vi "NMR only mode.vi"() -> ()   [LabVIEW 2010]
uses:
  QCA-Q_Curve_Acquisition/QCA Global.vi
panel:
  in  "setup\nfile":path=path "C:/Users/ptgroup/Documents/PDP/B28_Setup_File.txt"
  in  "DC convert":bool
  in  "DAC channel":u32
  in  "ADC channel":u32=1 step=1
  in  "Q meter number":u32=2 step=1
  out "update in (s)":u32
  in  "run":bool
  in  "single shot":bool
  in  "Yale gain":u16(ring)=1 items=["1", "20", "50"]
  in  "sweeps":u32=100
  in  "steps / second":u32=15287 step=1
  in  "steps":u32=500 step=1
  in  "amplitude (mV)":i32=275
  in  "modulation (kHz)":i32=400 step=1
  in  "center frequency (MHz)":dbl=213.0 min=0.0 step=0.001 format="%#_6f"
  out "NMR signal":cluster{dbl[], "Waveform Graph":dbl[]}(graph)
  # "RF settings"
  # "sweep settings"
  # "Q meter settings"
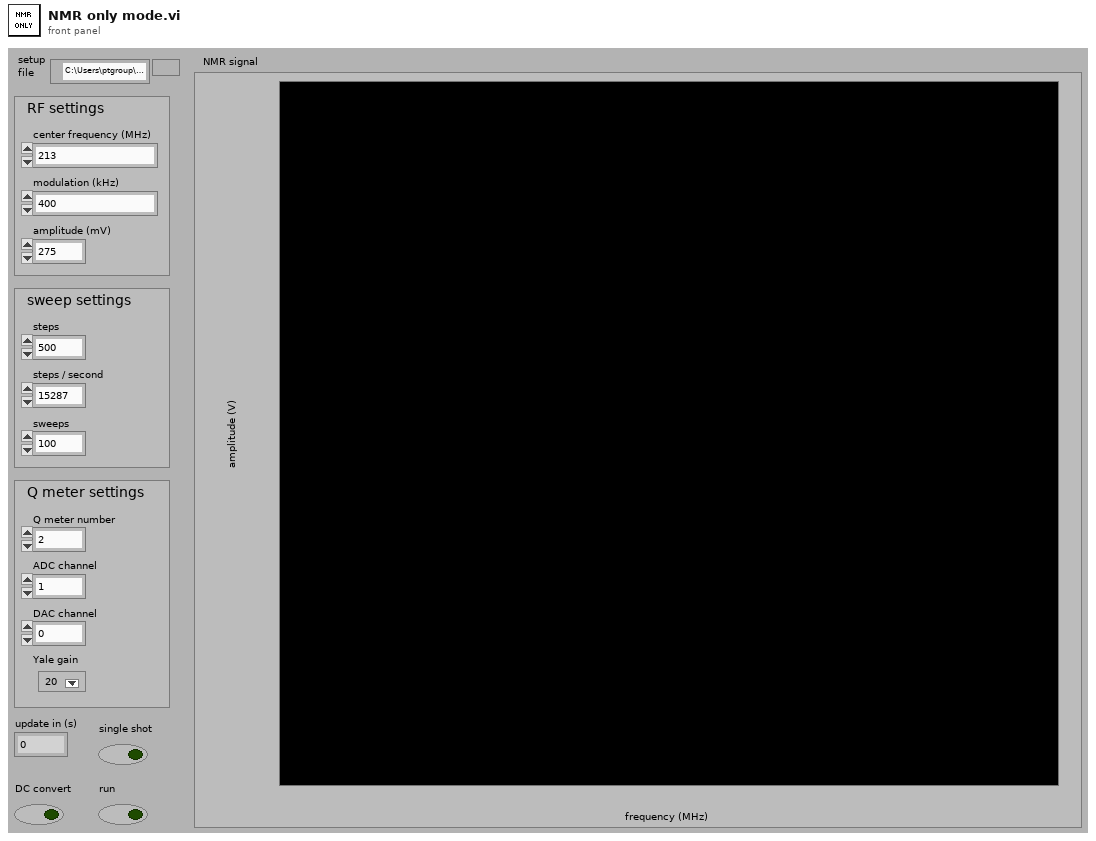
[diagram p1: front panel]
types:
  T1 = enum16{"initialize TPS", "initialize NMR", "initialize RF", "initialize Yale", "idle", "run", "single shot", "stop"}
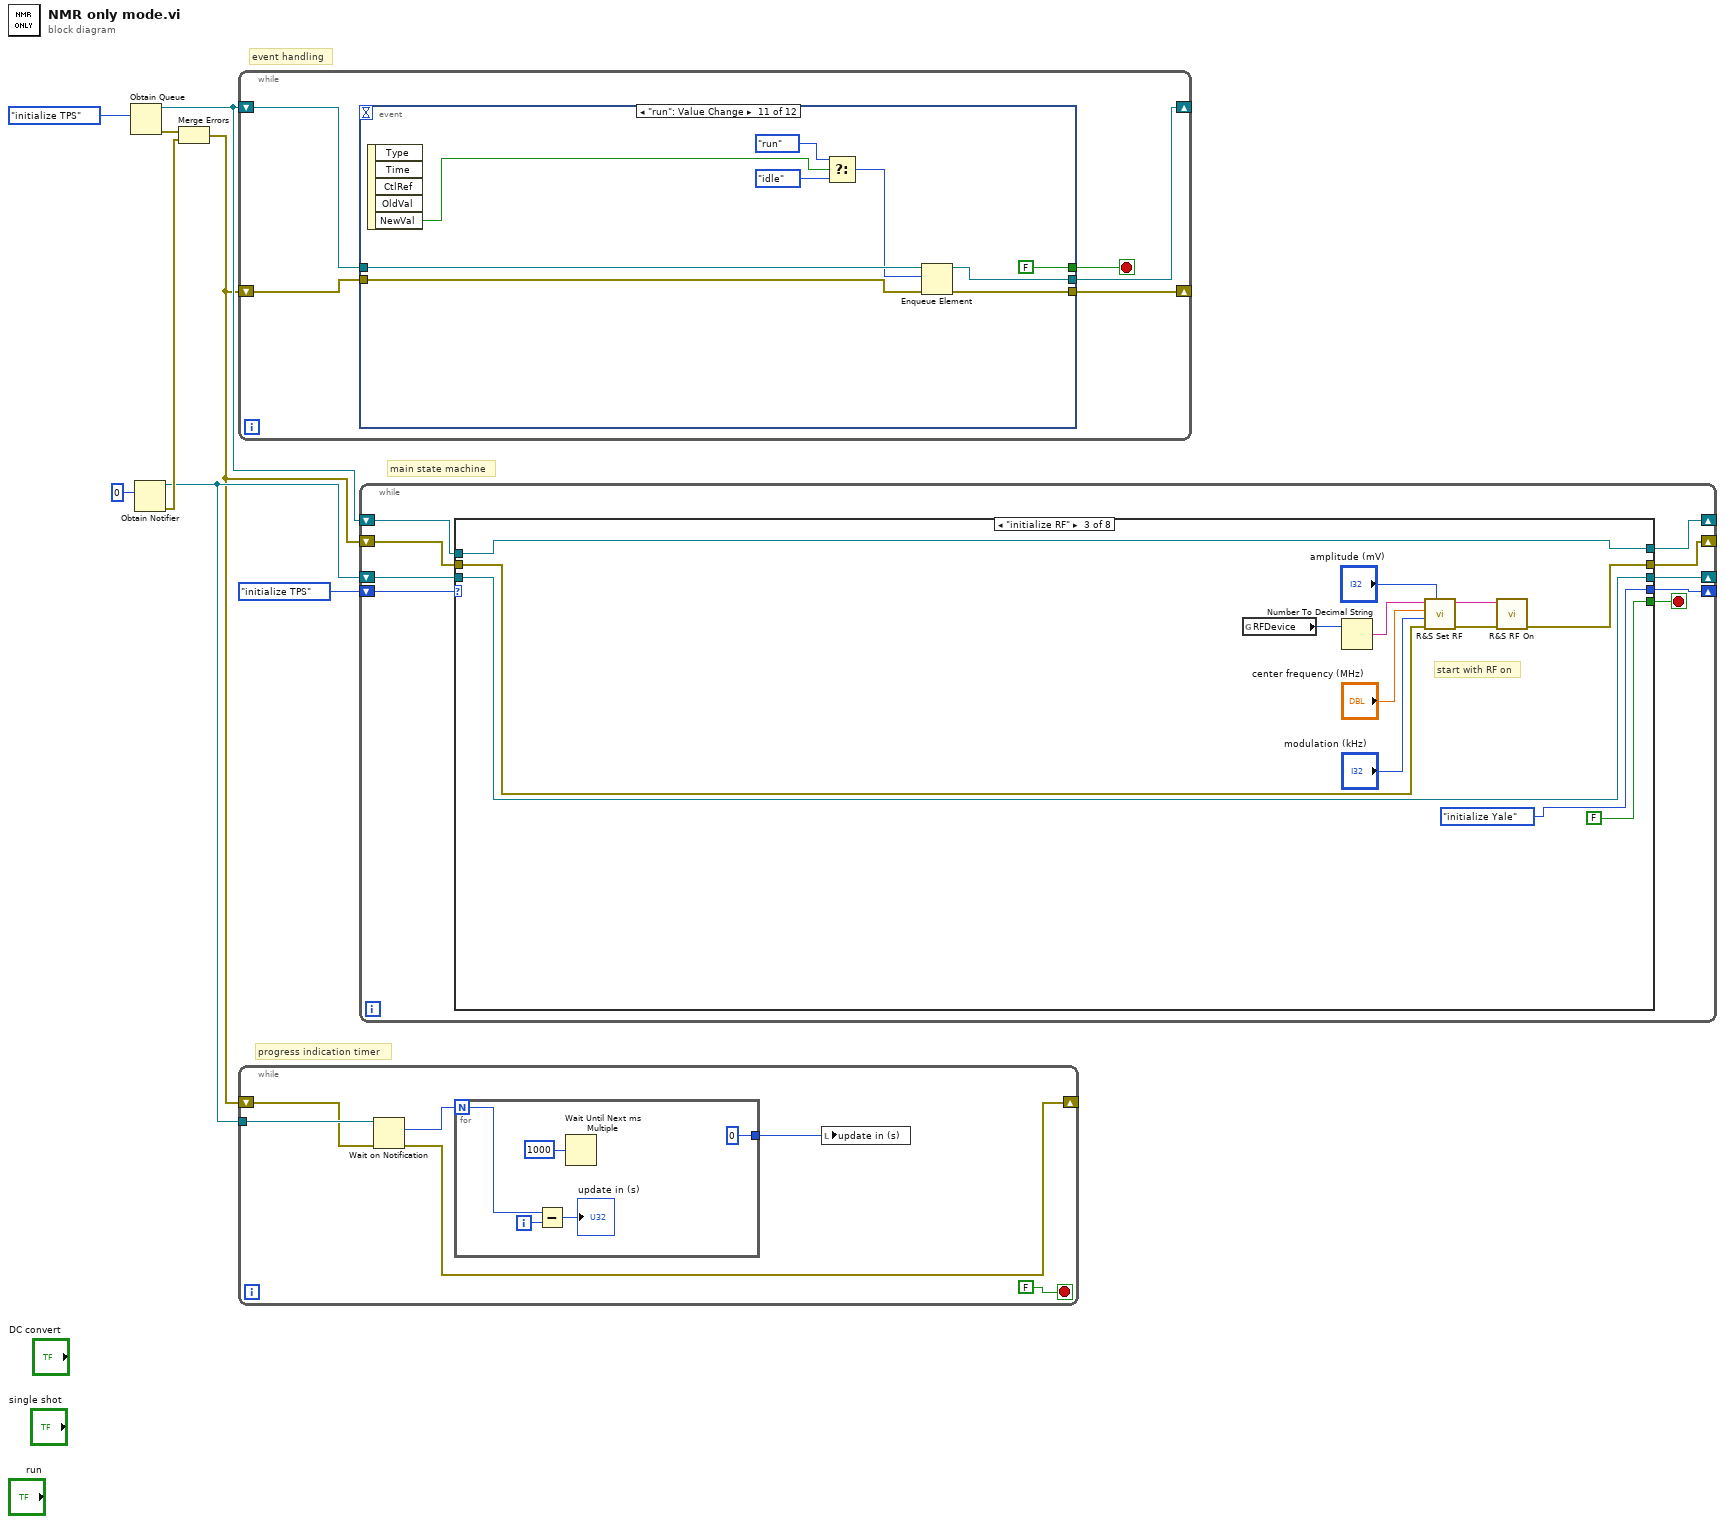
[diagram p0: block diagram]
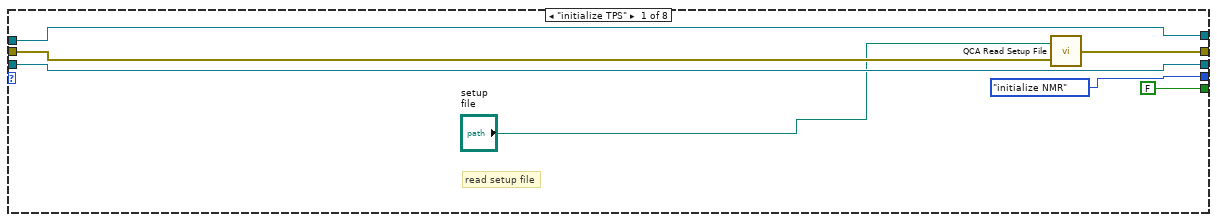
[diagram p2: hidden frame]
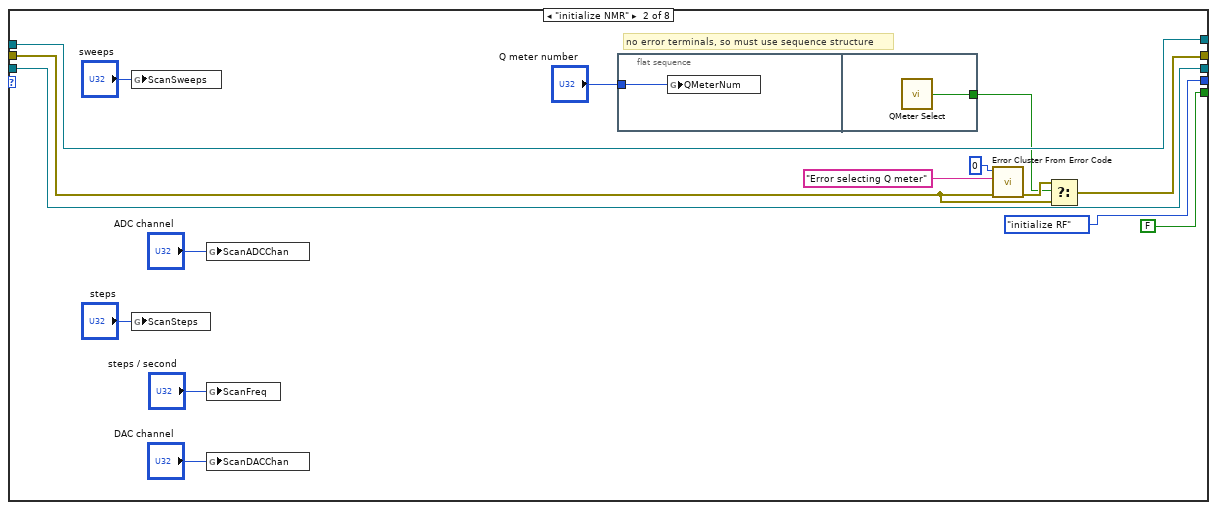
[diagram p3: hidden frame]
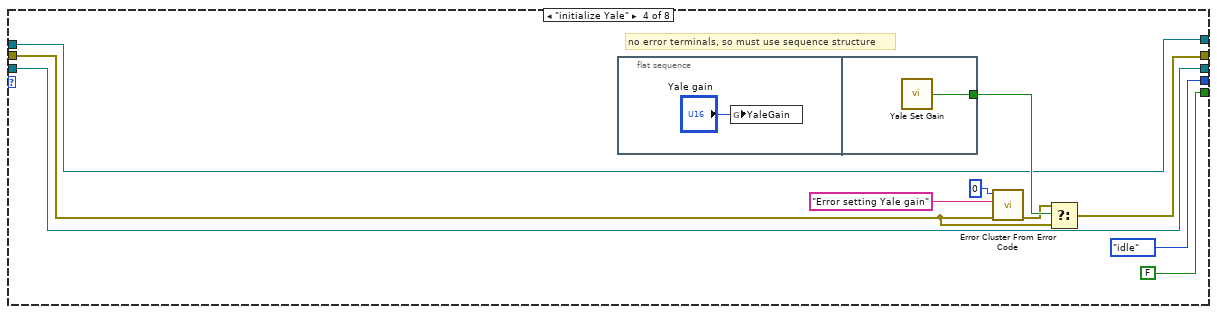
[diagram p4: hidden frame]
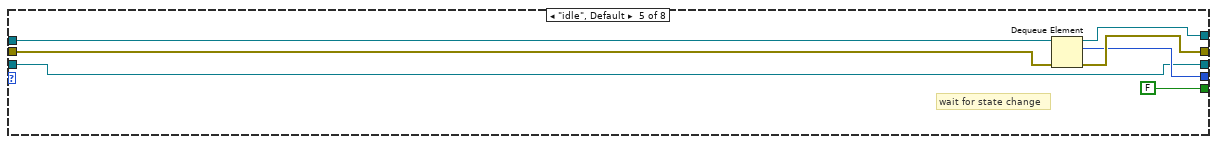
[diagram p5: hidden frame]
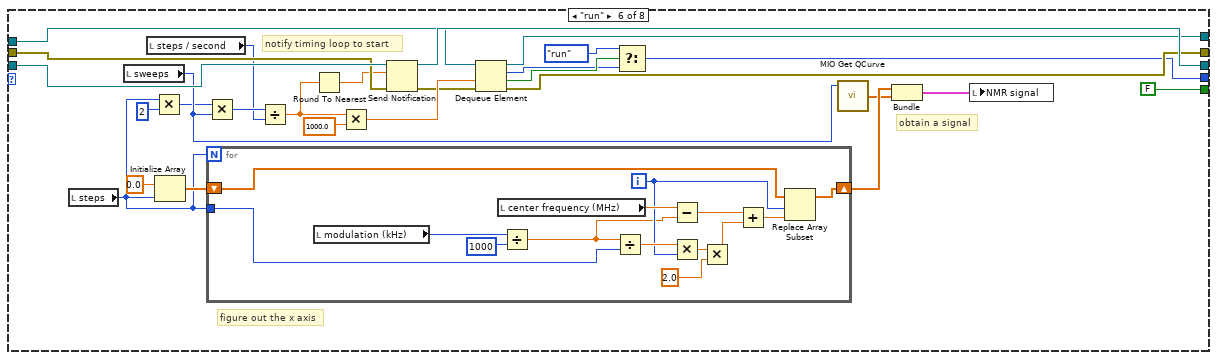
[diagram p6: hidden frame]
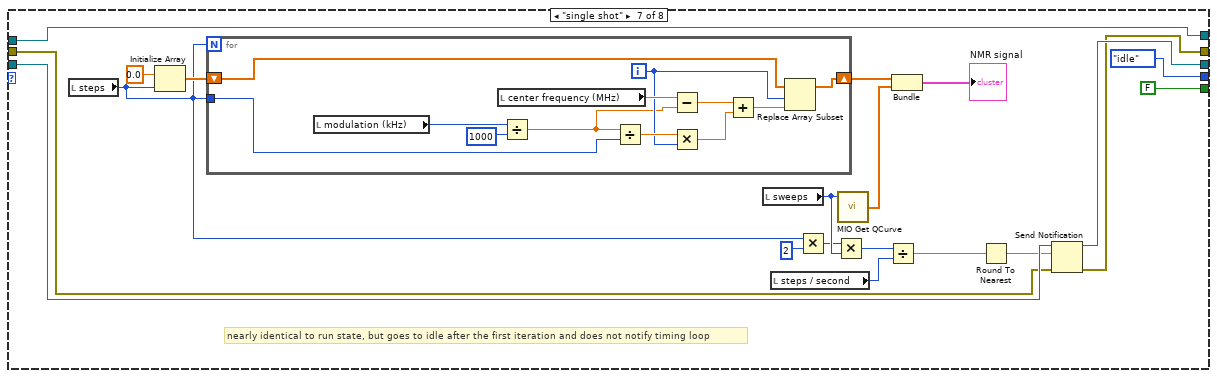
[diagram p7: hidden frame]
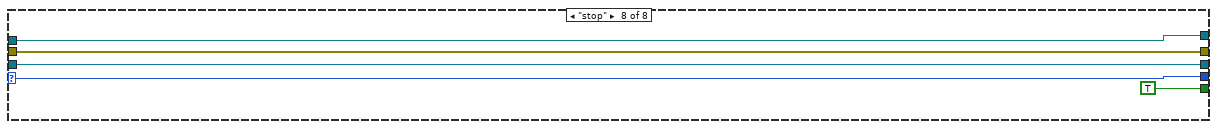
[diagram p8: hidden frame]
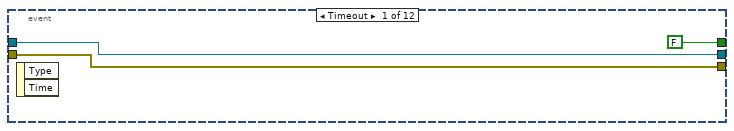
[diagram p9: hidden frame]
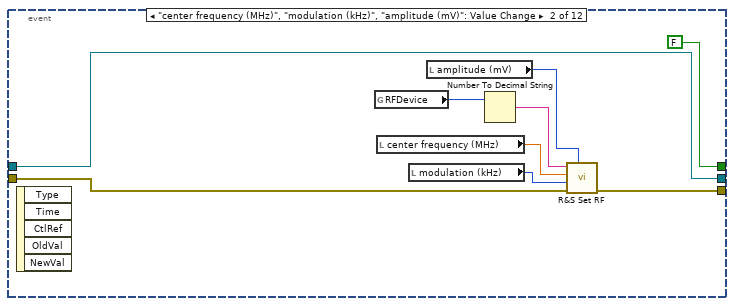
[diagram p10: hidden frame]
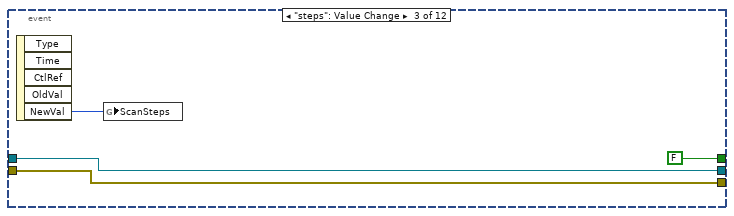
[diagram p11: hidden frame]
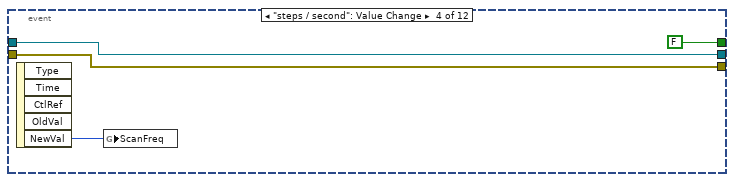
[diagram p12: hidden frame]
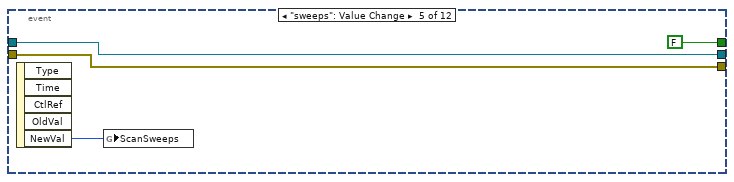
[diagram p13: hidden frame]
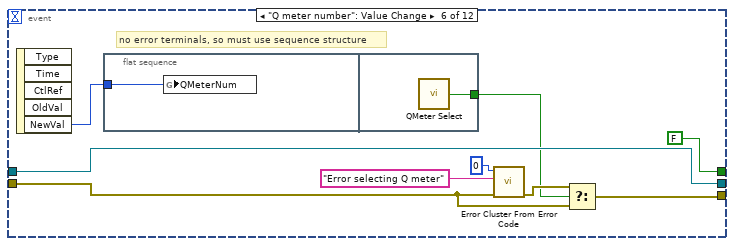
[diagram p14: hidden frame]
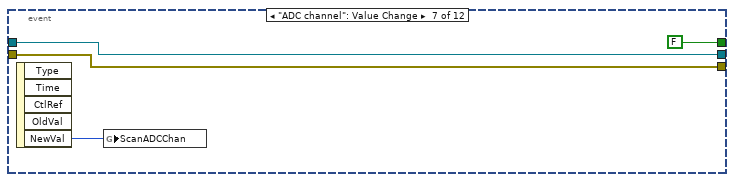
[diagram p15: hidden frame]
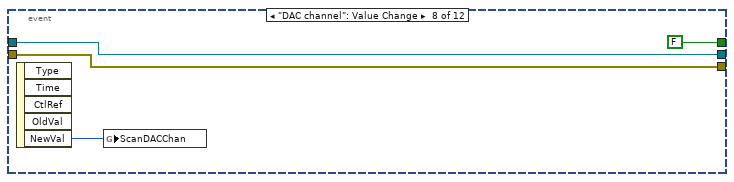
[diagram p16: hidden frame]
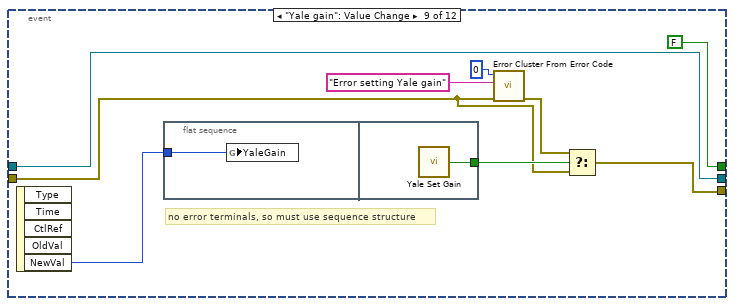
[diagram p17: hidden frame]
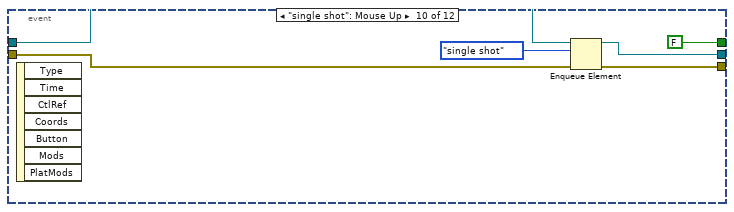
[diagram p18: hidden frame]
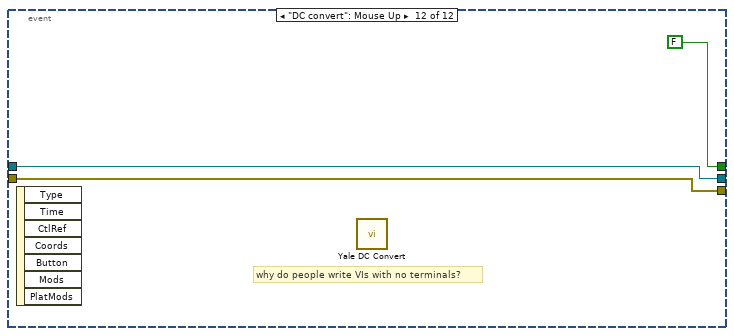
[diagram p19: hidden frame]
diagram:
  # "progress indication timer"
  # "main state machine"
  # "event handling"
  n1 = Obtain Queue(element data type=T1."initialize TPS") -> (queue out=w7:refnum<queue>, error out=w4:errorcluster)  [unwired: 4 in, 1 out]
  n2 = Obtain Notifier(notification data type=u32 0 ("update in (s)")) -> (notifier out=w2:refnum<notifier>, error out=w3:errorcluster)  [unwired: 3 in, 1 out]
  n3 = Merge Errors(w4, w3) -> (w1:errorcluster)
  n4 = while {
    shift-right: [w11] -> _
    shift-left: w1 -> [w12]
    shift-right: [w9] -> _
    shift-left: w7 -> [w10]
    stop <- w13 stop-if-true
    n5 = event shown="[10] \"run\": Value Change" {
      selector: _ -> [_ _ _ _ _ _ _ _ _ _ _ _]
      dyn-events: _ -> [_ _ _ _ _ _ _ _ _ _ _ _]
      timeout: _ -> [_ _ _ _ _ _ _ _ _ _ _ _]
      tunnel: [FALSE FALSE FALSE FALSE FALSE FALSE FALSE FALSE FALSE FALSE FALSE FALSE] -> w13
      tunnel: w12 -> [w15 w21 w27 w30 w34 w40 w49 w53 w60 w71 w80 w85]
      tunnel: [w15 w20 w27 w30 w34 w39 w49 w53 w62 w70 w79 w85] -> w11
      tunnel: w10 -> [w16 w24 w26 w31 w35 w45 w50 w54 w58 w73 w82 w83]
      tunnel: [w16 w24 w26 w31 w35 w45 w50 w54 w58 w72 w81 w83] -> w9
      event Timeout {
        n6 = event-data() -> ()  [unwired: 1 in, 2 out]
      }
      event "center frequency (MHz)", "modulation (kHz)", "amplitude (mV)": Value Change {
        n7 = event-data() -> ()  [unwired: 1 in, 5 out]
        n8 = global read "QCA Global.vi" "RFDevice"() -> (w18:i32)
        n9 = local read "center frequency (MHz)"() -> (w19:dbl)
        n10 = local read "modulation (kHz)"() -> (w23:i32)
        n11 = local read "amplitude (mV)"() -> (w22:i32)
        n12 = Number To Decimal String(number=w18) -> (decimal integer string=w17:string)  [unwired: 1 in]
        n13 = call "R&S Set RF.vi"("amplitude (mV)"=w22, "error in (no error)"=w21, "modulation (kHz)"=w23, "center frequency (MHz)"=w19, "address"=w17) -> ("error out"=w20:errorcluster)  [unwired: 2 in, 1 out]
      }
      event "steps": Value Change {
        n14 = event-data() -> ("NewVal"=w28:u32)  [unwired: 1 in, 4 out]
        n15 = global write "QCA Global.vi" "ScanSteps"(w28) -> ()
      }
      event "steps / second": Value Change {
        n16 = event-data() -> ("NewVal"=w32:u32)  [unwired: 1 in, 4 out]
        n17 = global write "QCA Global.vi" "ScanFreq"(w32) -> ()
      }
      event "sweeps": Value Change {
        n18 = event-data() -> ("NewVal"=w36:u32)  [unwired: 1 in, 4 out]
        n19 = global write "QCA Global.vi" "ScanSweeps"(w36) -> ()
      }
      event "Q meter number": Value Change {
        # "no error terminals, so must use sequence structure"
        n20 = event-data() -> ("NewVal"=w44:u32)  [unwired: 1 in, 4 out]
        n21 = flat-sequence {
          tunnel: w44 -> [w47]
          tunnel: [w48] -> w38
          frame #0 {
            n22 = global write "QCA Global.vi" "QMeterNum"(w47) -> ()
          }
          frame #1 {
            n23 = call "QMeter Select.vi"() -> ("Error"=w48:bool)
          }
        }
        n24 = call <vilib>:"Error Cluster From Error Code.vi"("error in (no error)"=w40, "error message (\"\")"="Error selecting Q meter" ("error message (\"\")"), "error code (0)"=0) -> ("error out"=w43:errorcluster)  [unwired: 6 in]
        n25 = Select(t=w43, s=w38, f=w40) -> (s? t:f=w39:errorcluster)
      }
      event "ADC channel": Value Change {
        n26 = event-data() -> ("NewVal"=w51:u32)  [unwired: 1 in, 4 out]
        n27 = global write "QCA Global.vi" "ScanADCChan"(w51) -> ()
      }
      event "DAC channel": Value Change {
        n28 = event-data() -> ("NewVal"=w55:u32)  [unwired: 1 in, 4 out]
        n29 = global write "QCA Global.vi" "ScanDACChan"(w55) -> ()
      }
      event "Yale gain": Value Change {
        # "no error terminals, so must use sequence structure"
        n30 = event-data() -> ("NewVal"=w65:u16)  [unwired: 1 in, 4 out]
        n31 = flat-sequence {
          tunnel: w65 -> [w66]
          tunnel: [w67] -> w63
          frame #0 {
            n32 = global write "QCA Global.vi" "YaleGain"(w66) -> ()
          }
          frame #1 {
            n33 = call "Yale Set Gain.vi"() -> ("Error"=w67:bool)
          }
        }
        n34 = call <vilib>:"Error Cluster From Error Code.vi"("error in (no error)"=w60, "error message (\"\")"="Error setting Yale gain" ("error message (\"\")"), "error code (0)"=0) -> ("error out"=w61:errorcluster)  [unwired: 6 in]
        n35 = Select(t=w61, s=w63, f=w60) -> (s? t:f=w62:errorcluster)
      }
      event "single shot": Mouse Up {
        n36 = event-data() -> ()  [unwired: 1 in, 7 out]
        n37 = Enqueue Element(queue=w73, element=T1."single shot", error in (no error)=w71) -> (queue out=w72:refnum<queue>, error out=w70:errorcluster)  [unwired: 1 in, 1 out]
      }
      event "run": Value Change {
        n38 = event-data() -> ("NewVal"=w77:bool)  [unwired: 1 in, 4 out]
        n39 = Select(t=T1."run", s=w77, f=T1."idle") -> (s? t:f=w76:T1)
        n40 = Enqueue Element(queue=w82, element=w76, error in (no error)=w80) -> (queue out=w81:refnum<queue>, error out=w79:errorcluster)  [unwired: 1 in, 1 out]
      }
      event "DC convert": Mouse Up {
        # "why do people write VIs with no terminals?"
        n41 = event-data() -> ()  [unwired: 1 in, 7 out]
        n42 = call "Yale DC Convert.vi"() -> ()  [unwired: 1 in]
      }
    }
  }
  n43 = while {
    tunnel: w2 -> [w90]
    shift-right: [w86] -> _
    shift-left: w1 -> [w89]
    stop <- FALSE stop-if-true
    n44 = Wait on Notification(notifier=w90, error in (no error)=w89) -> (notification=w88:u32, error out=w86:errorcluster)  [unwired: 2 in, 2 out]
    n45 = for {
      N: w88 -> [w96]
      tunnel: [0] -> w87
      i -> [w95]
      n46 = Subtract(x=w96, y=w95) -> (x-y=→"update in (s)":i32)
      n47 = Wait Until Next ms Multiple(millisecond multiple=u32 1000) -> ()  [unwired: 1 out]
    }
    n48 = local write "update in (s)"(w87) -> ()
  }
  n49 = while {
    shift-right: [w103] -> _
    shift-left: w7 -> [w104]
    shift-right: [w101] -> _
    shift-left: w1 -> [w102]
    shift-right: [w100] -> _
    shift-left: T1."initialize TPS" -> [w105]
    shift-right: [w98] -> _
    shift-left: w2 -> [w99]
    stop <- w97 stop-if-true
    n50 = case shown="\"initialize RF\"" w105 {
      selector: w105 -> [_ _ _ _ _ _ _ w239]
      tunnel: w104 -> [w112 w128 w143 w148 w161 w179 w223 w240]
      tunnel: [w112 w128 w143 w148 w162 w172 w223 w240] -> w103
      tunnel: w102 -> [w108 w114 w136 w149 w156 w188 w221 w237]
      tunnel: [w107 w113 w133 w150 w160 w173 w208 w237] -> w101
      tunnel: [T1."initialize NMR" T1."initialize RF" T1."initialize Yale" T1."idle" w159 w171 T1."idle" w239] -> w100
      tunnel: w99 -> [w110 w121 w132 w146 w158 w189 w222 w238]
      tunnel: [w110 w121 w132 w146 w158 w185 w216 w238] -> w98
      tunnel: [FALSE FALSE FALSE FALSE FALSE FALSE FALSE TRUE] -> w97
      frame "initialize TPS" {
        # "read setup file"
        n51 = call "QCA Read Setup File.vi"("error in (no error)"=w108, "setup file"="setup\nfile") -> ("error out"=w107:errorcluster)
      }
      frame "initialize NMR" {
        # "no error terminals, so must use sequence structure"
        n52 = global write "QCA Global.vi" "ScanSweeps"("sweeps") -> ()
        n53 = global write "QCA Global.vi" "ScanSteps"("steps") -> ()
        n54 = global write "QCA Global.vi" "ScanADCChan"("ADC channel") -> ()
        n55 = global write "QCA Global.vi" "ScanFreq"("steps / second") -> ()
        n56 = global write "QCA Global.vi" "ScanDACChan"("DAC channel") -> ()
        n57 = flat-sequence {
          tunnel: "Q meter number" -> [w129]
          tunnel: [w130] -> w116
          frame #0 {
            n58 = global write "QCA Global.vi" "QMeterNum"(w129) -> ()
          }
          frame #1 {
            n59 = call "QMeter Select.vi"() -> ("Error"=w130:bool)
          }
        }
        n60 = call <vilib>:"Error Cluster From Error Code.vi"("error in (no error)"=w114, "error message (\"\")"="Error selecting Q meter" ("error message (\"\")"), "error code (0)"=0) -> ("error out"=w119:errorcluster)  [unwired: 6 in]
        n61 = Select(t=w119, s=w116, f=w114) -> (s? t:f=w113:errorcluster)
      }
      frame "initialize RF" {
        # "start with RF on"
        n62 = global read "QCA Global.vi" "RFDevice"() -> (w140:i32)
        n63 = Number To Decimal String(number=w140) -> (decimal integer string=w139:string)  [unwired: 1 in]
        n64 = call "R&S Set RF.vi"("amplitude (mV)"="amplitude (mV)", "error in (no error)"=w136, "modulation (kHz)"="modulation (kHz)", "center frequency (MHz)"="center frequency (MHz)", "address"=w139) -> ("error out"=w134:errorcluster, "address out"=w135:string)  [unwired: 2 in]
        n65 = call "R&S RF On.vi"("error in (no error)"=w134, "address"=w135) -> ("error out"=w133:errorcluster)  [unwired: 4 in, 1 out]
      }
      frame "initialize Yale" {
        # "no error terminals, so must use sequence structure"
        n66 = flat-sequence {
          tunnel: [w155] -> w152
          frame #0 {
            n67 = global write "QCA Global.vi" "YaleGain"("Yale gain") -> ()
          }
          frame #1 {
            n68 = call "Yale Set Gain.vi"() -> ("Error"=w155:bool)
          }
        }
        n69 = call <vilib>:"Error Cluster From Error Code.vi"("error in (no error)"=w149, "error message (\"\")"="Error setting Yale gain" ("error message (\"\")"), "error code (0)"=0) -> ("error out"=w151:errorcluster)  [unwired: 6 in]
        n70 = Select(t=w151, s=w152, f=w149) -> (s? t:f=w150:errorcluster)
      }
      frame "idle", Default {
        # "wait for state change"
        n71 = Dequeue Element(queue=w161, error in (no error)=w156) -> (queue out=w162:refnum<queue>, element=w159:T1, error out=w160:errorcluster)  [unwired: 1 in, 1 out]
      }
      frame "run" {
        # "obtain a signal"
        # "notify timing loop to start"
        # "figure out the x axis"
        n72 = local read "steps"() -> (w165:u32)
        n73 = local read "sweeps"() -> (w184:u32)
        n74 = local read "steps / second"() -> (w186:u32)
        n75 = Multiply(x=w165, y=u32 2) -> (x*y=w164:u32)
        n76 = Initialize Array(0.0 ("element"), w165) -> (w182:dbl[])
        n77 = Multiply(x=w164, y=w184) -> (x*y=w187:u32)
        n78 = for {
          N: w165 -> [_]
          shift-right: [w194] -> w181
          shift-left: w182 -> [w203]
          tunnel: w165 -> [w199]
          i -> [w196]
          n79 = local read "modulation (kHz)"() -> (w198:i32)
          n80 = local read "center frequency (MHz)"() -> (w202:dbl)
          n81 = Divide(x=w198, y=u32 1000) -> (x/y=w193:dbl)
          n82 = Divide(x=w193, y=w199) -> (x/y=w197:dbl)
          n83 = Subtract(x=w202, y=w193) -> (x-y=w200:dbl)
          n84 = Multiply(x=w197, y=w196) -> (x*y=w192:dbl)
          n85 = Multiply(x=w192, y=2.0) -> (x*y=w191:dbl)
          n86 = Add(x=w200, y=w191) -> (x+y=w195:dbl)
          n87 = Replace Array Subset(array=w203, new element=w195, index=w196) -> (w194:dbl[])
        }
        n88 = Divide(x=w187, y=w186) -> (x/y=w176:dbl)
        n89 = Round To Nearest(number=w176) -> (nearest integer value=w178:dbl)
        n90 = Multiply(x=w176, y=1000.0) -> (x*y=w175:dbl)
        n91 = Send Notification(notification=w178, notifier=w189, error in (no error)=w188) -> (notifier out=w185:refnum<notifier>, error out=w174:errorcluster)
        n92 = Dequeue Element(queue=w179, timeout in ms (-1)=w175, error in (no error)=w174) -> (queue out=w172:refnum<queue>, element=w168:T1, timed out?=w170:bool, error out=w173:errorcluster)
        n93 = Select(t=T1."run", s=w170, f=w168) -> (s? t:f=w171:T1)
        n94 = call "MIO Get QCurve.vi"("Num Sweeps"=w184) -> ("Waveform Graph"=w180:dbl[])  [unwired: 2 in]
        n95 = Bundle(w181, "Waveform Graph"=w180) -> (w167:cluster{dbl[], "Waveform Graph":dbl[]})  [unwired: 1 in]
        n96 = local write "NMR signal"(w167) -> ()
      }
      frame "single shot" {
        # "nearly identical to run state, but goes to idle after the first iteration and does not notify timing loop"
        n97 = local read "steps"() -> (w206:u32)
        n98 = Initialize Array(0.0 ("element"), w206) -> (w213:dbl[])
        n99 = for {
          N: w206 -> [_]
          shift-right: [w226] -> w212
          shift-left: w213 -> [w235]
          tunnel: w206 -> [w231]
          i -> [w228]
          n100 = local read "modulation (kHz)"() -> (w230:i32)
          n101 = local read "center frequency (MHz)"() -> (w234:dbl)
          n102 = Divide(x=w230, y=u32 1000) -> (x/y=w225:dbl)
          n103 = Divide(x=w225, y=w231) -> (x/y=w229:dbl)
          n104 = Subtract(x=w234, y=w225) -> (x-y=w232:dbl)
          n105 = Multiply(x=w229, y=w228) -> (x*y=w224:dbl)
          n106 = Add(x=w232, y=w224) -> (x+y=w227:dbl)
          n107 = Replace Array Subset(array=w235, new element=w227, index=w228) -> (w226:dbl[])
        }
        n108 = local read "sweeps"() -> (w215:u32)
        n109 = local read "steps / second"() -> (w219:u32)
        n110 = Multiply(x=w206, y=u32 2) -> (x*y=w205:u32)
        n111 = Multiply(x=w205, y=w215) -> (x*y=w220:u32)
        n112 = call "MIO Get QCurve.vi"("Num Sweeps"=w215) -> ("Waveform Graph"=w211:dbl[])  [unwired: 2 in]
        n113 = Divide(x=w220, y=w219) -> (x/y=w218:dbl)
        n114 = Bundle(w212, "Waveform Graph"=w211) -> (→"NMR signal":cluster{dbl[], "Waveform Graph":dbl[]})  [unwired: 1 in]
        n115 = Round To Nearest(number=w218) -> (nearest integer value=w217:dbl)
        n116 = Send Notification(notification=w217, notifier=w222, error in (no error)=w221) -> (notifier out=w216:refnum<notifier>, error out=w208:errorcluster)
      }
      frame "stop" {
      }
    }
  }
